vi "Robot.vi"() -> ()   [LabVIEW 2013]
uses:
  <vilib>/Utility/inputDevices.llb/closeJoystick.vi
  <vilib>/Utility/inputDevices.llb/joystickAcquire.vi
  <vilib>/Utility/file.llb/Write To Spreadsheet File (DBL).vi
  <vilib>/ptbypt/NI_PtbyPt.lvlib
panel:
  out "mAh":dbl
  out "Hopper Open":bool
  out "Distance From Bin":dbl
  out "?":dbl
  out "Actuator 2":dbl(slide) scale=0.0..1005.0
  out "?":dbl
  out "Actuator 1":dbl(slide) scale=0.0..1005.0
  out "?":dbl
  out "Pulley Current":dbl(slide) scale=0.0..30.0
  out "BAT 9":bool
  out "BAT 8":bool
  out "BAT 7":bool
  out "BAT 6":bool
  out "DataLog":bool
  out "SysMsg":bool
  out "Array":dbl[][](array[numeric])
  out "Total Power":dbl
  out "Inst Power":dbl
  out "Avg Power":dbl
  out "?":dbl
  out "BLCurrent":dbl(slide) scale=0.0..30.0
  out "A":dbl
  out "?":dbl
  out "?":dbl
  out "Volts":dbl
  out "Amps":dbl
  out "BAT 5":bool
  out "BAT 3":bool
  out "BAT 2":bool
  out "Main Current":dbl(knob) scale=0.0..30.0
  out "connection ID 2":refnum<k5>
  out "JoyStick String with CheckSum":string
  in  "Simulate error 2":bool
  in  "Simulate error":bool
  out "BR Current":dbl(slide) scale=0.0..30.0
  out "FL Current":dbl(slide) scale=0.0..30.0
  out "FR Current":dbl(slide) scale=0.0..30.0
  in  "Joystick Loop":bool
  out "SysMsg 2":refnum<file>
  out "Datalog":refnum<file>
  in  "Boolean 3":bool
  out "Outgoing Strings":string
  out "System Messages":string
  out "Elapsed Time":timestamp format="%<%M:%S%3u>T"
  in  "Reset":bool
  out "SysMsg":refnum<file>
  out "BAT":bool
  out "Battery":dbl(slide) scale=0.0..100.0
  in  "TX cue Loop":bool
  out "Trigger":i8
  out "Dpad":i32
  out "Buttons":bool[](array[boolean])
  out "Bytes Written":i32
  out "Boolean 2":bool
  in  "WDT Loop":bool
  in  "WDT Reset":bool caption="Reset"
  out "WDT (s)":dbl caption="Elapsed Time (s)"
  out "WDT expired":bool caption="Time has Elapsed"
  out "HB":bool
  in  "ALL STOP":bool
  out "error out":errorcluster
  in  "Reconnect":bool
  out "Incoming Strings":string
  out "Connected":bool
  in  "local host":bool
  out "connection ID":refnum<k5>
  out "Main Voltage":dbl(knob) scale=0.0..16.0
  # "ALARM"
  # "NETWORK"
  # "Battery"
  # "POWER"
  # "FILE IO"
  # "WATCHDOG"
  # "CONTROL"
  # "%"
  # "Power"
  # "Error Panel"
  # "W"
  # "W"
  # "W"
  # "time remaining"
  # "Motor Currents"
  # "LINEAR ACTUATORS"
  # "In"
  # "A"
  # "A"
  # "A"
  # "A"
types:
  T1 = enum16{"open", "replace", "create", "open or create", "replace or create", "replace or create with confirmation"}
  T2 = enum16{"Standard", "Buffered", "CRLF", "Immediate"}
  T3 = cluster{"unsigned byte array[0]":u8, "unsigned byte array[1]":u8, "unsigned byte array[2]":u8, "unsigned byte array[3]":u8, "unsigned byte array[4]":u8, "unsigned byte array[5]":u8, "unsigned byte array[6]":u8, "unsigned byte array[7]":u8, "unsigned byte array[8]":u8}
  T4 = cluster{"X axis":i32, "Y axis":i32, "Z axis":i32, "X axis rotation":i32, "Y axis rotation":i32, "Z axis rotation":i32, "U axis":i32, "V axis":i32}
  T5 = cluster{"button 1":bool, "button 2":bool, "button 3":bool, "button 4":bool, "button 5":bool, "button 6":bool, "button 7":bool, "button 8":bool, "button 9":bool, "button 10":bool, "button 11":bool, "button 12":bool, "button 13":bool, "button 14":bool, "button 15":bool, "button 16":bool, "button 17":bool, "button 18":bool, "button 19":bool, "button 20":bool, "button 21":bool, "button 22":bool, "button 23":bool, "button 24":bool, "button 25":bool, "button 26":bool, "button 27":bool, "button 28":bool, "button 29":bool, "button 30":bool, "button 31":bool, "button 32":bool}
  T6 = cluster{"pov 1":i32, "pov 2":i32, "pov 3":i32, "pov 4":i32}
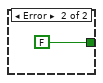
[diagram p2: hidden frame]
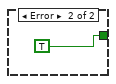
[diagram p3: hidden frame]
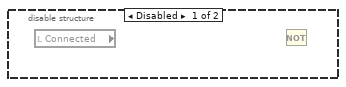
[diagram p11: hidden frame]
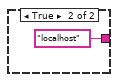
[diagram p12: hidden frame]
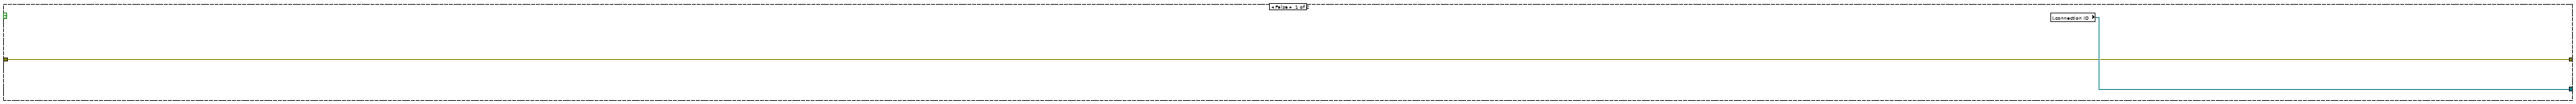
[diagram p15: hidden frame]
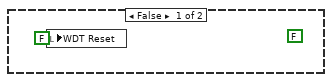
[diagram p16: hidden frame]
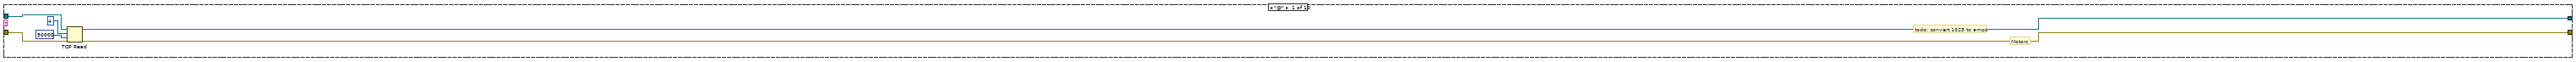
[diagram p17: hidden frame]
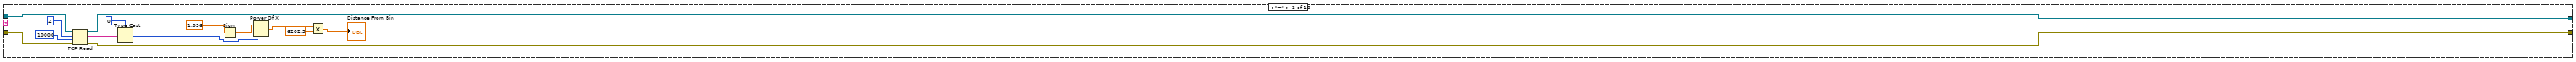
[diagram p18: hidden frame]
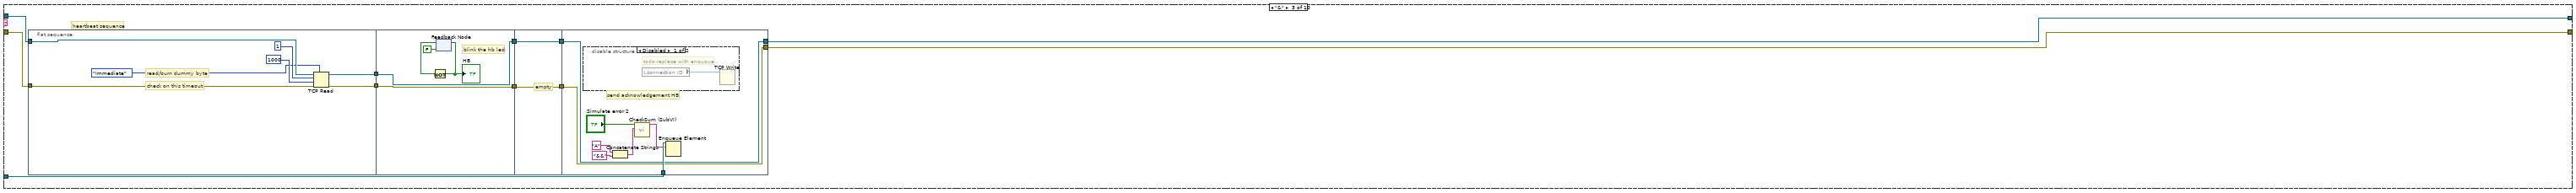
[diagram p19: hidden frame]
diagram:
  # "press main loop stop button to write \ncollected pwr data to this file"
  # "Location of collected power data"
  # "Global/ Holds the Connection state"
  # "Message cue loop"
  # "setup the log file"
  # "Setup the system message file, will auto replace"
  # "create a cue"
  n1 = while {
    stop <- "WDT Loop" stop-if-true
    # "tell us when we reconnect"
    # "when wdtexp goes from false\nto true, we will write a\nsystem msg saying \nlabview wdt timed out"
    # "show time we've been disconnected"
    # "signal (local)"
    # "MAIN CLOCK"
    # "WATCHDOG AND MAIN CLOCK LOOP"
    # "auto reset is disabled"
    # "local bool"
    # "wtd timout (s)"
    # "WATCHDOG"
    n2 = disable-structure shown="Enabled" {
      frame Disabled {
        n3 = local read "Connected"() -> (w50:bool)
        n4 = Not() -> ()  [unwired: 1 in, 1 out]
      }
      frame Enabled {
      }
    }
    n5 = case shown="True" "Boolean 3" {
      frame False {
      }
      frame True {
        n6 = call "Elapsed Time2"("Reset"="Reset", "Auto Reset"=FALSE) -> ("Elapsed Time (s)"=w48:dbl)  [unwired: 10 in, 7 out]
        n7 = To Time Stamp(1:w48) -> (0:→"Elapsed Time":timestamp)
      }
    }
    n8 = local read "WDT Reset"() -> (w38:bool)
    n9 = call "Elapsed Time"("Time Target (s)"=0.75, "Reset"=w38, "Auto Reset"=FALSE) -> ("Elapsed Time (s)"=→"WDT (s)":dbl, "Time has Elapsed"=w30:bool)  [unwired: 9 in, 6 out]
    "WDT expired" <- w30
    n10 = call <vilib>:"Boolean Crossing PtByPt.vi"("direction"=enum16{"either", "false-true", "true-false"}."true-false", "input"=w30) -> ("crossing"=w29:bool)  [unwired: 1 in]
    n11 = case shown="True" w29 {
      frame False {
      }
      frame True {
        n12 = local read "Elapsed Time"() -> (w40:timestamp)
        n13 = local read "SysMsg"() -> (w42:refnum<file>)
        n14 = call "Alarm (SubVI).vi"("String"="LV Watchdog reset", "Elapsed Time"=w40, "Byte Stream File in"=w42) -> ()  [unwired: 8 in, 1 out]
      }
    }
    n15 = call <vilib>:"Boolean Crossing PtByPt.vi"("direction"=enum16{"either", "false-true", "true-false"}."false-true", "input"=w30) -> ("crossing"=w32:bool)  [unwired: 1 in]
    n16 = case shown="True" w32 {
      frame False {
      }
      frame True {
        n17 = local read "Elapsed Time"() -> (w45:timestamp)
        n18 = local read "SysMsg"() -> (w43:refnum<file>)
        n19 = call "Alarm (SubVI).vi"("String"="LV Watchdog timeout", "Elapsed Time"=w45, "Byte Stream File in"=w43) -> ()  [unwired: 8 in, 1 out]
      }
    }
  }
  n20 = Obtain Queue(element data type="") -> (queue out=w7:refnum<queue>)  [unwired: 4 in, 2 out]
  n21 = Build Path(base path=path "C:/robot/branches/Nick/Robot" ("App:Default Data Directory"), name or relative path="log.txt") -> (appended path=w10:path)
  n22 = Build Path(base path=path "C:/robot/branches/Nick/Robot" ("App:Default Data Directory"), name or relative path="SysMsg.txt") -> (appended path=w13:path)
  n23 = while {
    tunnel: [w58] -> w28
    tunnel: [w57] -> w27
    tunnel: w7 -> [w52]
    tunnel: ["ALL STOP"] -> w6
    stop <- "ALL STOP" stop-if-true
    # "RECEIVE LOOP + non-time critical tasks"
    n24 = flat-sequence {
      tunnel: [w62] -> w53
      tunnel: [w74] -> w54
      tunnel: w53 -> [w74]
      tunnel: [w76] -> w60
      tunnel: [w75] -> w55
      tunnel: w54 -> [w75]
      tunnel: w60 -> [w82]
      tunnel: [w81] -> w59
      tunnel: [w80] -> w56
      tunnel: w55 -> [w79]
      tunnel: w52 -> [w78]
      tunnel: w59 -> [w341]
      tunnel: [w340] -> w58
      tunnel: [w339] -> w57
      tunnel: w56 -> [w335]
      frame #0 {
      }
      frame #1 {
        # "reconnect routine"
        # "2 tcp connect if not connected (also performs reconnect)"
        n25 = local read "Connected"() -> (w63:bool)
        n26 = case shown="False" w63 {
          tunnel: [w68 _] -> w62
          tunnel: "local host" -> [w65 _]
          frame False {
            # "reset wdt?"
            n27 = case shown="False" w65 {
              tunnel: ["192.168.1.50" ("address") "localhost"] -> w64
              frame False {
              }
              frame True {
              }
            }
            n28 = TCP Open Connection(address=w64, remote port or service name=u16 2000, timeout ms (60000)=50) -> (connection ID=→"connection ID":refnum<k5>, error out=w68:errorcluster)  [unwired: 2 in]
          }
          frame True {
          }
        }
        "Boolean 2" <- "local host"
      }
      frame #2 {
        # "UPDATE System Messages"
        n29 = call "Last5lines (SubVI).vi"("File Path Control"=path "C:/robot/branches/Nick/Robot/SysMsg.txt") -> ("Output"=→"System Messages":string)  [unwired: 7 in, 3 out]
      }
      frame #3 {
        # "this code needs to be fixec"
        # "4 if we didnt write anything, \nwe are not connected?"
        # "if connected"
        # "instead of 1 i think this shoud \nconnect to wtd expired instead?"
        n30 = disable-structure shown="Enabled" {
          frame Disabled {
          }
          frame Enabled {
          }
        }
        n31 = Not Equal To 0?(x=1 ("Bytes Written")) -> (x != 0?=w76:bool)
        n32 = local write "Connected"(w76) -> ()
      }
      frame #4 {
        # "5 read incoming bytes, else N/C"
        n33 = case shown="True" w82 {
          tunnel: [w84 w85] -> w81
          tunnel: [w83 w86] -> w80
          tunnel: w79 -> [w83 w89]
          tunnel: w78 -> [_ w88]
          frame False {
            n34 = local read "connection ID"() -> (w84:refnum<k5>)
          }
          frame True {
            # "global variable"
            # "step 1:"
            # "Handle Incoming message case statement"
            # "Reset is local"
            # "message id"
            # "not in use (yet)"
            # "reset the watchdog timer"
            # "if we recieved\nsomething..."
            # "read 1 byte(id byte)"
            # "note: this timeout \nis important to \nthe watchdog, \nmaybe should be less"
            # "pass message id into switch case --->"
            n35 = local read "connection ID"() -> (w92:refnum<k5>)
            n36 = TCP Read(connection ID=w92, bytes to read=1, error in (no error)=w89, 7:T2."Immediate" ("mode (standard)"), 9:600 ("timeout ms (25000)")) -> (connection ID out=w94:refnum<k5>, data out=w91:string, error out=w93:errorcluster)
            "Incoming Strings" <- w91
            n37 = case shown="\"V\"" w91 {
              tunnel: w94 -> [w105 w119 w129 w167 w176 w186 w198 w254 w277 w317]
              tunnel: w93 -> [w102 w118 w130 w168 w177 w184 w201 w253 w276 w316]
              tunnel: [w101 w112 w127 w165 w177 w183 w199 w255 w266 w295] -> w86
              tunnel: w88 -> [_ _ w124 _ _ _ _ _ _ _]
              tunnel: [w100 w113 w123 w164 w176 w185 w200 w232 w267 w296] -> w85
              frame "@" {
                # "todo: convert 1023 to amps"
                # "Motors"
                n38 = TCP Read(connection ID=w105, bytes to read=4, error in (no error)=w102, 9:50000 ("timeout ms (25000)")) -> (connection ID out=w100:refnum<k5>, error out=w101:errorcluster)  [unwired: 1 in, 1 out]
              }
              frame "~" {
                n39 = TCP Read(connection ID=w119, bytes to read=2, error in (no error)=w118, 9:10000 ("timeout ms (25000)")) -> (connection ID out=w113:refnum<k5>, data out=w115:string, error out=w112:errorcluster)  [unwired: 1 in]
                n40 = Type Cast(type=u16 0, x=w115) -> (*(type *) &x=w109:u16)
                n41 = Sign(1:1.056) -> (0:w110:dbl)
                n42 = Power Of X(1:w109, 2:w110) -> (0:w108:dbl)
                n43 = Multiply(x=w108, y=6202.3) -> (x*y=→"Distance From Bin":dbl)
              }
              frame "&" {
                # "heartbeat sequence"
                n44 = flat-sequence {
                  tunnel: w130 -> [w135]
                  tunnel: w129 -> [w134]
                  tunnel: [w133] -> w128
                  tunnel: [w131] -> w120
                  tunnel: [w139] -> w126
                  tunnel: w128 -> [w139]
                  tunnel: [w138] -> w121
                  tunnel: w120 -> [w138]
                  tunnel: w126 -> [w144]
                  tunnel: [w144] -> w125
                  tunnel: [w143] -> w122
                  tunnel: w121 -> [w143]
                  tunnel: w125 -> [w151]
                  tunnel: [w151] -> w127
                  tunnel: w124 -> [w152]
                  tunnel: [w150] -> w123
                  tunnel: w122 -> [w150]
                  frame #0 {
                    # "check on this timeout"
                    # "read/burn dummy byte"
                    n45 = TCP Read(connection ID=w134, bytes to read=1, error in (no error)=w135, 7:T2."Immediate" ("mode (standard)"), 9:1000 ("timeout ms (25000)")) -> (connection ID out=w131:refnum<k5>, error out=w133:errorcluster)  [unwired: 1 out]
                  }
                  frame #1 {
                    # "blink the hb led"
                    n46 = feedback #1(FALSE) -> (w141:bool)
                    n47 = Not(x=w141) -> (.not. x?=w140:bool)
                    "HB" <- w140
                    n48 = feedback-in #1(w140) -> ()
                  }
                  frame #2 {
                    # "empty"
                  }
                  frame #3 {
                    # "send acknowledgement HB"
                    n49 = disable-structure shown="Disabled" {
                      frame Disabled {
                        # "todo:replace with enquque"
                        n50 = local read "connection ID"() -> (w153:refnum<k5>)
                        n51 = TCP Write(connection ID=w153) -> ()  [unwired: 3 in, 3 out]
                      }
                      frame Enabled {
                      }
                    }
                    n52 = Concatenate Strings("A" ("data in"), "&&" ("string")) -> (w147:string)
                    n53 = call "CheckSum (SubVI).vi"("String"=w147, "Simulate error"="Simulate error 2") -> ("string"=w145:string)  [unwired: 8 in, 1 out]
                    n54 = Enqueue Element(queue=w152, element=w145) -> ()  [unwired: 2 in, 3 out]
                  }
                }
              }
              frame "^" {
                # "calc bin angle,\nconnect to this indicator"
                # "check on this timeout"
                # "read/burn dummy byte"
                n55 = TCP Read(connection ID=w167, bytes to read=4, error in (no error)=w168, 7:T2."Immediate" ("mode (standard)"), 9:1000 ("timeout ms (25000)")) -> (connection ID out=w164:refnum<k5>, data out=w166:string, error out=w165:errorcluster)
                n56 = String To Byte Array(string=w166) -> (unsigned byte array=w163:u8[])
                n57 = Array To Cluster(array=w163) -> (cluster=w162:T3)
                n58 = Unbundle By Name(w162) -> ("unsigned byte array[0]"=w161:u8, "unsigned byte array[1]"=w160:u8, "unsigned byte array[2]"=w159:u8, "unsigned byte array[3]"=w158:u8)
                n59 = Join Numbers(hi=w159, lo=w158) -> ((hi.lo)=w154:u16)
                "Actuator 2" <- w154
                "?" <- w154
                n60 = Join Numbers(hi=w161, lo=w160) -> ((hi.lo)=w157:u16)
                "Actuator 1" <- w157
                "?" <- w157
                n61 = Greater Or Equal?(x=w157, y=u16 1000) -> (x >= y?=w155:bool)
                n62 = case shown="False" w155 {
                  tunnel: w154 -> [_ w174]
                  frame False {
                    n63 = local write "Hopper Open"(FALSE) -> ()
                  }
                  frame True {
                    n64 = Greater Or Equal?(x=w174, y=u16 1000) -> (x >= y?=w173:bool)
                    n65 = local write "Hopper Open"(w173) -> ()
                  }
                }
              }
              frame "*", Default {
                # "wifly hello (or something)"
                # "this is often system messages from wifly"
              }
              frame "!" {
                w188 = u16 1  # u16
                # "todo: write to log also"
                # "update sys"
                # "send ACK"
                # "alarm code"
                # "alarm lookup"
                # "ALARM"
                # "alarm case structure"
                n66 = TCP Read(connection ID=w186, bytes to read=2, error in (no error)=w184, 9:1000 ("timeout ms (25000)")) -> (connection ID out=w185:refnum<k5>, data out=w189:string, error out=w183:errorcluster)  [unwired: 1 in]
                n67 = Type Cast(type=w188, x=w189) -> (*(type *) &x=w179:u16)
                n68 = call "Alarm Lookup (SubVI).vi"("Alarm Code"=w179) -> ("Alarm Meaning"=w180:string)  [unwired: 10 in]
                n69 = local read "Elapsed Time"() -> (w181:timestamp)
                n70 = local read "SysMsg"() -> (w182:refnum<file>)
                n71 = call "Alarm (SubVI).vi"("String"=w180, "Elapsed Time"=w181, "Byte Stream File in"=w182) -> ("Alarm Indicator"=w178:bool)  [unwired: 8 in]
                n72 = case shown="3" w179 {
                  tunnel: w178 -> [_ w191]
                  frame 0, Default {
                  }
                  frame 3 {
                    "BAT 3" <- w191
                  }
                }
              }
              frame "%" {
                # "not used yet"
                # "not in use currently"
                n73 = TCP Read(connection ID=w198, bytes to read=1, error in (no error)=w201, 9:1000 ("timeout ms (25000)")) -> (connection ID out=w200:refnum<k5>, data out=w197:string, error out=w199:errorcluster)  [unwired: 1 in]
                n74 = Type Cast(type=u8 0, x=w197) -> (*(type *) &x=w195:u8)
                n75 = call "RobotStateLookUp(SubVI).vi"("Numeric"=w195) -> ("element"=w194:string)  [unwired: 10 in]
                n76 = local read "Elapsed Time"() -> (w193:timestamp)
                n77 = local read "SysMsg"() -> (w192:refnum<file>)
                n78 = call "RobotStateWrite (SubVI).vi"("time stamp"=w193, "string"=w194, "Byte Stream File in"=w192) -> ()  [unwired: 9 in]
              }
              frame "V" {
                # "to hrs"
                # "to mins"
                # "get mAh  consumed for battery calcs"
                # "convert to from mAsecs"
                # "Current"
                # "POWER STUFF"
                # "this calculates and displays all power calculations (in real time) and also stores  this data for later use in an array.\nThe pwr data in the array is written to a text file when we press the main loop stop button on the VI after our run is over."
                # "% out"
                # "max battery level (volts)"
                # "alarm"
                # "Voltage"
                # "convert to Voltage"
                # "split the battery voltage off to the battery monitor section"
                # "check for low battery"
                # "-->"
                # "todo: convert 1023 eq to float voltage"
                # "battery voltage"
                # "current battery level (volts)"
                # "min battery level (volts)"
                # "read another 2 bytes"
                n79 = TCP Read(connection ID=w254, bytes to read=4, error in (no error)=w253, 9:50000 ("timeout ms (25000)")) -> (connection ID out=w232:refnum<k5>, data out=w248:string, error out=w255:errorcluster)  [unwired: 1 in]
                n80 = String To Byte Array(string=w248) -> (unsigned byte array=w247:u8[])
                n81 = Array To Cluster(array=w247) -> (cluster=w246:T3)
                n82 = Unbundle By Name(w246) -> ("unsigned byte array[0]"=w220:u8, "unsigned byte array[1]"=w219:u8, "unsigned byte array[2]"=w244:u8, "unsigned byte array[3]"=w243:u8)
                n83 = Join Numbers(hi=w220, lo=w219) -> ((hi.lo)=w245:u16)
                n84 = Join Numbers(hi=w244, lo=w243) -> ((hi.lo)=w242:u16)
                n85 = To Word Integer(number=w245) -> (16bit integer=w218:i16)
                n86 = To Unsigned Word Integer(number=w242) -> (unsigned 16bit integer=w241:u16)
                n87 = Subtract(x=w218, y=i16 163) -> (x-y=w216:i16)
                n88 = call "MainVandCur(SubVI).vi"("Main CurrentADC"=w241) -> ("Current Out"=w212:dbl)  [unwired: 9 in, 1 out]
                "Main Current" <- w212
                "Amps" <- w212
                n89 = call "MainVandCur(SubVI).vi"("Main Voltage ADC"=w216) -> ("Voltage out"=w224:dbl)  [unwired: 9 in, 1 out]
                "Main Voltage" <- w224
                "Volts" <- w224
                n90 = Multiply(x=w212, y=1000.0) -> (x*y=w210:dbl)
                n91 = Divide(x=w210, y=60.0) -> (x/y=w208:dbl)
                n92 = Divide(x=w208, y=60.0) -> (x/y=w206:dbl)
                n93 = feedback #2(0.0) -> (w215:dbl)
                n94 = Add(x=w215, y=w206) -> (x+y=w213:dbl)
                "mAh" <- w213
                n95 = feedback-in #2(w213) -> ()
                n96 = Multiply(x=w224, y=w212) -> (x*y=w223:dbl)
                "Inst Power" <- w223
                n97 = feedback #3(0.0) -> (w234:dbl)
                n98 = Add(x=w234, y=w223) -> (x+y=w221:dbl)
                n99 = Divide(x=w221, y=1000.0) -> (x/y=→"Total Power":dbl)
                n100 = feedback-in #3(w221) -> ()
                n101 = feedback #4(0.0) -> (w236:dbl)
                n102 = Increment(x=w236) -> (x+1=w237:dbl)
                n103 = Divide(x=w221, y=w237) -> (x/y=w222:dbl)
                "Avg Power" <- w222
                n104 = feedback-in #4(w237) -> ()
                n105 = call "Battery Percentage (SubVI).vi"("Battery Voltage"=w224, "Min Battery Voltage"=9.6 ("y"), "Max Battery Voltage"=12.4 ("x")) -> ("Battery Percent Remaining"=w239:dbl)  [unwired: 8 in]
                "Battery" <- w239
                n106 = call "Elapsed Time3"("Time Target (s)"=20.0, "Set Start Time (s)"=0.0) -> ("Elapsed Time (s)"=w225:dbl)  [unwired: 10 in, 7 out]
                n107 = Build Array(w225, w224, w212, w223, w222, w221) -> (w228:dbl[])
                n108 = Less?(x=w239, y=30.0) -> (x < y?=w249:bool)
                n109 = Less Or Equal?(x=w239, y=4.0) -> (x <= y?=w240:bool)
                n110 = case shown="True" w249 {
                  frame False {
                  }
                  frame True {
                    n111 = local read "Elapsed Time"() -> (w262:timestamp)
                    n112 = local read "SysMsg"() -> (w264:refnum<file>)
                    n113 = call "Alarm (SubVI).vi"("String"="Battery Low", "Elapsed Time"=w262, "Byte Stream File in"=w264) -> ("Alarm Indicator"=→"BAT":bool)  [unwired: 8 in]
                  }
                }
                n114 = feedback #5(dbl[][] []) -> (w231:dbl[][])
                "Array" <- w231
                n115 = case shown="True" w240 {
                  frame False {
                  }
                  frame True {
                    n116 = local read "Elapsed Time"() -> (w260:timestamp)
                    n117 = local read "SysMsg"() -> (w259:refnum<file>)
                    n118 = call "Alarm (SubVI).vi"("String"="Battery Critical", "Elapsed Time"=w260, "Byte Stream File in"=w259) -> ("Alarm Indicator"=→"BAT 2":bool)  [unwired: 8 in]
                  }
                }
                n119 = Build Array (concatenate)(w231, w228) -> (w229:dbl[][])
                n120 = feedback-in #5(w229) -> ()
              }
              frame "P" {
                n121 = TCP Read(connection ID=w277, bytes to read=2, error in (no error)=w276, 9:25000 ("timeout ms (25000)")) -> (connection ID out=w267:refnum<k5>, data out=w273:string, error out=w266:errorcluster)  [unwired: 1 in]
                n122 = Type Cast(type=u16 0, x=w273) -> (*(type *) &x=w271:u16)
                n123 = call "mtrADCtoAmps(SubVI).vi"("ADCcurrent"=w271) -> ("Numeric"=w270:dbl)  [unwired: 10 in]
                "?" <- w270
                "Pulley Current" <- w270
                n124 = Equal?(x=w270, y=0.0) -> (x = y?=w268:bool)
                n125 = case shown="True" w268 {
                  frame False {
                  }
                  frame True {
                    n126 = local read "Elapsed Time"() -> (w279:timestamp)
                    n127 = local read "SysMsg"() -> (w278:refnum<file>)
                    n128 = call "Alarm (SubVI).vi"("String"="Power Failuer On Pulley", "Elapsed Time"=w279, "Byte Stream File in"=w278) -> ("Alarm Indicator"=→"BAT 9":bool)  [unwired: 8 in]
                  }
                }
              }
              frame "C" {
                # "do power calcs?"
                # "main current"
                # "alarms + lookup"
                n129 = TCP Read(connection ID=w317, bytes to read=8, error in (no error)=w316, 9:1000 ("timeout ms (25000)")) -> (connection ID out=w296:refnum<k5>, data out=w300:string, error out=w295:errorcluster)  [unwired: 1 in]
                n130 = String To Byte Array(string=w300) -> (unsigned byte array=w314:u8[])
                n131 = Array To Cluster(array=w314) -> (cluster=w313:T3)
                n132 = Unbundle By Name(w313) -> ("unsigned byte array[0]"=w312:u8, "unsigned byte array[1]"=w311:u8, "unsigned byte array[2]"=w309:u8, "unsigned byte array[3]"=w308:u8, "unsigned byte array[4]"=w306:u8, "unsigned byte array[5]"=w305:u8, "unsigned byte array[6]"=w303:u8, "unsigned byte array[7]"=w302:u8)
                n133 = Join Numbers(hi=w312, lo=w311) -> ((hi.lo)=w310:u16)
                n134 = Join Numbers(hi=w309, lo=w308) -> ((hi.lo)=w307:u16)
                n135 = Join Numbers(hi=w306, lo=w305) -> ((hi.lo)=w304:u16)
                n136 = Join Numbers(hi=w303, lo=w302) -> ((hi.lo)=w301:u16)
                n137 = To Unsigned Word Integer(number=w310) -> (unsigned 16bit integer=w294:u16)
                n138 = To Unsigned Word Integer(number=w307) -> (unsigned 16bit integer=w299:u16)
                n139 = To Unsigned Word Integer(number=w304) -> (unsigned 16bit integer=w298:u16)
                n140 = To Unsigned Word Integer(number=w301) -> (unsigned 16bit integer=w297:u16)
                n141 = call "mtrADCtoAmps(SubVI).vi"("ADCcurrent"=w299) -> ("Numeric"=w293:dbl)  [unwired: 10 in]
                "FR Current" <- w293
                "?" <- w293
                n142 = call "mtrADCtoAmps(SubVI).vi"("ADCcurrent"=w298) -> ("Numeric"=w288:dbl)  [unwired: 10 in]
                "FL Current" <- w288
                "?" <- w288
                n143 = call "mtrADCtoAmps(SubVI).vi"("ADCcurrent"=w297) -> ("Numeric"=w285:dbl)  [unwired: 10 in]
                "BR Current" <- w285
                "A" <- w285
                n144 = call "mtrADCtoAmps(SubVI).vi"("ADCcurrent"=w294) -> ("Numeric"=w283:dbl)  [unwired: 10 in]
                "BLCurrent" <- w283
                "?" <- w283
                n145 = Equal?(x=w285, y=0.0) -> (x = y?=w284:bool)
                n146 = Equal?(x=w293, y=0.0) -> (x = y?=w291:bool)
                n147 = Equal?(x=w283, y=0.0) -> (x = y?=w282:bool)
                n148 = Equal?(x=w288, y=0.0) -> (x = y?=w287:bool)
                n149 = case shown="True" w282 {
                  frame False {
                  }
                  frame True {
                    n150 = local read "SysMsg"() -> (w320:refnum<file>)
                    n151 = local read "Elapsed Time"() -> (w319:timestamp)
                    n152 = call "Alarm (SubVI).vi"("String"="Power Failure BL", "Elapsed Time"=w319, "Byte Stream File in"=w320) -> ("Alarm Indicator"=→"BAT 8":bool)  [unwired: 8 in]
                  }
                }
                n153 = case shown="True" w287 {
                  frame False {
                  }
                  frame True {
                    n154 = local read "Elapsed Time"() -> (w327:timestamp)
                    n155 = local read "SysMsg"() -> (w328:refnum<file>)
                    n156 = call "Alarm (SubVI).vi"("String"="Power Failure FL", "Elapsed Time"=w327, "Byte Stream File in"=w328) -> ("Alarm Indicator"=→"BAT 6":bool)  [unwired: 8 in]
                  }
                }
                n157 = case shown="True" w284 {
                  frame False {
                  }
                  frame True {
                    n158 = local read "Elapsed Time"() -> (w324:timestamp)
                    n159 = local read "SysMsg"() -> (w323:refnum<file>)
                    n160 = call "Alarm (SubVI).vi"("String"="Power Failure BR", "Elapsed Time"=w324, "Byte Stream File in"=w323) -> ("Alarm Indicator"=→"BAT 7":bool)  [unwired: 8 in]
                  }
                }
                n161 = case shown="True" w291 {
                  frame False {
                  }
                  frame True {
                    n162 = local read "Elapsed Time"() -> (w332:timestamp)
                    n163 = local read "SysMsg"() -> (w331:refnum<file>)
                    n164 = call "Alarm (SubVI).vi"("String"="Power Failure FR", "Elapsed Time"=w332, "Byte Stream File in"=w331) -> ("Alarm Indicator"=→"BAT 5":bool)  [unwired: 8 in]
                  }
                }
              }
            }
            n165 = String Length(string=w91) -> (length=w90:i32)
            n166 = Greater Than 0?(x=w90) -> (x > 0?=w87:bool)
            n167 = case shown="True" w87 {
              frame False {
                (unwired) FALSE
                n168 = local write "WDT Reset"(FALSE) -> ()
              }
              frame True {
                n169 = local write "WDT Reset"(TRUE) -> ()
              }
            }
          }
        }
      }
      frame #5 {
        # "WDT expired indicator"
        # "manual reconnect button"
        # "if reconnect is pushed or the watchdog has expired, connected becomes false, tcp closes, and the loop starts again with no connection and therefore will attempt to re-connect"
        n170 = local read "WDT expired"() -> (w336:bool)
        n171 = Or(x=w336, y="Reconnect") -> (x .or. y?=w337:bool)
        n172 = case shown="True" w337 {
          tunnel: w341 -> [w343 w347]
          tunnel: [w342 w346] -> w339
          tunnel: [w343 w345] -> w340
          tunnel: w335 -> [w342 w344]
          frame False {
          }
          frame True {
            n173 = local write "Connected"(FALSE ("Connection Active?")) -> ()
            n174 = TCP Close Connection(connection ID=w347, error in (no error)=w344) -> (connection ID out=w345:refnum<k5>, error out=w346:errorcluster)  [unwired: 1 in]
          }
        }
      }
    }
  }
  n175 = while {
    tunnel: w7 -> [w357]
    stop <- "TX cue Loop" stop-if-true
    # "todo: \nif joystick id\nif it's new button press\nwhile ACK payload != joystick byte5chksm\nsend joystick again every 100ms\nexit on 400ms timeout(alarm), or ACK\ncontinue  with cue"
    # "write the message"
    # "decue next message"
    # "OUTGOING MESSAGE CUE LOOP"
    n176 = Dequeue Element(queue=w357) -> (element=w349:string)  [unwired: 2 in, 3 out]
    n177 = Wait (ms)(milliseconds to wait=u32 13) -> ()  [unwired: 1 out]
    n178 = local read "connection ID"() -> (w355:refnum<k5>)
    n179 = Concatenate Strings("$" ("string"), w349, "*") -> (w351:string)
    "Outgoing Strings" <- w351
    n180 = TCP Write(connection ID=w355, data in=w351) -> (bytes written=→"Bytes Written":i32, error out=w354:errorcluster)  [unwired: 2 in, 1 out]
    n181 = case shown="Error" w354 {
      frame No Error {
      }
      frame Error {
      }
    }
  }
  n182 = Open/Create/Replace File(file path (use dialog)=w10) -> (refnum out=→"Datalog":refnum<file>, error out=w4:errorcluster)  [unwired: 5 in, 1 out]
  n183 = Open/Create/Replace File(file path (use dialog)=w13, operation (0:open)=T1."replace or create") -> (refnum out=→"SysMsg":refnum<file>, error out=w3:errorcluster)  [unwired: 4 in, 1 out]
  n184 = case shown="No Error" w3 {
    tunnel: [FALSE ("BAT 6") TRUE ("BAT 6")] -> w2
    frame No Error {
    }
    frame Error {
    }
  }
  "SysMsg" <- w2
  n185 = case shown="No Error" w4 {
    tunnel: [FALSE FALSE ("DataLog")] -> w1
    frame No Error {
    }
    frame Error {
    }
  }
  "DataLog" <- w1
  n186 = call <vilib>:"Query Input Devices.vi"() -> ("error out"=w23:errorcluster)  [unwired: 1 in, 10 out]
  n187 = call <vilib>:"Initialize Joystick.vi"("error in (no error)"=w23, "device index"=4) -> ("error out"=w21:errorcluster, "device ID"=w22:refnum<k1>)  [unwired: 8 out]
  n188 = while {
    tunnel: w22 -> [w371]
    tunnel: w21 -> [w370]
    tunnel: [w369] -> w20
    tunnel: [w368] -> w19
    shift-right: [w365] -> _
    shift-left: _ -> [w366]
    tunnel: w7 -> [w364]
    stop <- "Joystick Loop" stop-if-true
    # "JOYSTCK/KEYBOARD POLLING LOOP"
    n189 = flat-sequence {
      tunnel: w371 -> [w381]
      tunnel: w370 -> [w380]
      tunnel: [w379] -> w369
      tunnel: [w378] -> w368
      tunnel: [w372] -> w367
      tunnel: w367 -> [w406]
      tunnel: w366 -> [w407]
      tunnel: [w406] -> w365
      tunnel: w364 -> [w405]
      frame #0 {
        # "ID"
        # "display"
        # "put them into 1 byte"
        # "assemble all joystick data into string"
        # "1 read the joystick"
        # "trigger buttons"
        # "dpad"
        # "reg buttons"
        n190 = call-poly <vilib>:"Acquire Input Data.vi"("device ID"=w381, "error in (no error)"=w380) -> ("device ID"=w378:refnum<k1>, "axis info"=w401:T4, "button info"=w389:T5, "direction info"=w385:T6, "error out"=w379:errorcluster)  [unwired: 13 out]
        n191 = Unbundle By Name(w389) -> ("button 1"=w390:bool, "button 2"=w391:bool, "button 3"=w392:bool, "button 4"=w393:bool, "button 5"=w394:bool, "button 6"=w395:bool, "button 7"=w396:bool, "button 8"=w397:bool)
        n192 = Unbundle By Name(w401) -> ("Z axis"=w400:i32)
        n193 = call "scale (SubVI).vi"("data"=w400) -> ("output"=w403:i8)  [unwired: 4 in]
        "Trigger" <- w403
        n194 = Build Array(w390, w391, w392, w393, w394, w395, w396, w397) -> (w377:bool[])
        "Buttons" <- w377
        n195 = Boolean Array To Number(Boolean array=w377) -> (number=w398:u32)
        n196 = To Unsigned Byte Integer(number=w398) -> (unsigned 8bit integer=w383:u8)
        n197 = Unbundle By Name(w385) -> ("pov 1"=w386:i32)
        "Dpad" <- w386
        n198 = To Word Integer(number=w386) -> (16bit integer=w387:i16)
        n199 = Not(x=w383) -> (.not. x?=w384:u8)
        n200 = Type Cast(x=w387) -> (*(type *) &x=w399:string)  [unwired: 1 in]
        n201 = Type Cast(x=w403) -> (*(type *) &x=w402:string)  [unwired: 1 in]
        n202 = Type Cast(x=w384) -> (*(type *) &x=w382:string)  [unwired: 1 in]
        n203 = Concatenate Strings("#" ("string"), w382, w399, w402) -> (w375:string)
        n204 = call "CheckSum (SubVI).vi"("String"=w375, "Simulate error"="Simulate error") -> ("Numeric"=w374:u8)  [unwired: 8 in, 1 out]
        n205 = Type Cast(x=w374) -> (*(type *) &x=w373:string)  [unwired: 1 in]
        n206 = Concatenate Strings(w375, w373) -> (w372:string)
        "JoyStick String with CheckSum" <- w372
      }
      frame #1 {
        # "if true send/if false dont send"
        # "previous message"
        # "if this new message \nis the same as the \nprev one we just sent \nthen dont send it"
        # "save the last thing we sent"
        # "3 write joystick only when something changes"
        n207 = Not Equal?(x=w407, y=w406) -> (x != y?=w404:bool)
        n208 = case shown="True" w404 {
          tunnel: w405 -> [_ w409]
          frame False {
          }
          frame True {
            n209 = local read "JoyStick String with CheckSum"() -> (w408:string)
            n210 = disable-structure shown="Enabled" {
              frame Disabled {
              }
              frame Enabled {
              }
            }
            n211 = Enqueue Element(queue=w409, element=w408) -> ()  [unwired: 2 in, 3 out]
          }
        }
      }
    }
  }
  n212 = call-poly <vilib>:"Close Input Device.vi"("error in (no error)"=w20, "device ID"=w19) -> ("error out"=w18:errorcluster)  [unwired: 8 out]
  n213 = TCP Close Connection(connection ID=w28, error in (no error)=w27) -> (error out=w26:errorcluster)  [unwired: 1 in, 1 out]
  n214 = Merge Errors(w26, w18) -> (w25:errorcluster)
  "error out" <- w25
  n215 = call <vilib>:"General Error Handler.vi"("error in (no error)"=w25) -> ()  [unwired: 1 in, 14 out]
  n216 = case shown="True" w6 {
    tunnel: path "C:/robot/branches/Nick/Robot/Pwr_Data.txt" ("start path") -> [_ w411]
    frame False {
    }
    frame True {
      n217 = local read "Array"() -> (w410:dbl[][])
      n218 = call-poly <vilib>:"Write To Spreadsheet File.vi"("format (%.3f)"="%.3f", "2D data"=w410, "file path (dialog if empty)"=w411) -> ()  [unwired: 5 in, 1 out]
    }
  }
